vi "GrabCallBackThread_FullFeatures.vi"(11 "Error IN":errorcluster) -> (15 "Error OUT":errorcluster)   [LabVIEW 2014]
uses:
  <vilib>/addons/PixeLINK/Low Level Functions/TRANSLATION.llb/TDPU-Translation-CallBackFlags.ctl
  <vilib>/addons/PixeLINK/Low Level Functions/TRANSLATION.llb/TDPU-Translation-CallbacksInfo.ctl
  <vilib>/addons/PixeLINK/Low Level Functions/ACQUISITION.llb/TDPU-Acquisition-Frame_Desc.ctl
  <vilib>/addons/PixeLINK/Low Level Functions/TRANSLATION.llb/TDPU-Translation-PixelFormat.ctl
  <vilib>/addons/PixeLINK/Low Level Functions/ACQUISITION.llb/TDPU-Acquisition-StreamState.ctl
  <vilib>/addons/PixeLINK/Low Level Functions/CAMERA_FEATURES.llb/TDPU-CameraFeatures-FeatureIds.ctl
  <vilib>/addons/PixeLINK/Low Level Functions/CAMERA_FEATURES.llb/TDPU-CameraFeatures-FeatureFlags.ctl
  PxLLabVIEW.dll
panel:
  in  "Trig":u16(ring) items=["Freerun", "Software", "Hardware"]
  in  "Stop Processing Events":bool
  out "Loop info":string
  in  "Exposure time":dbl=7e-05 min=7e-05 max=5.0
  out "Intensity Graph":u16[][](graph)
  out "Frame Number":u32
  out "Missed Frames":u32
  out "FrameData_FORMAT":T1 items=["PIXEL_FORMAT_MONO8", "PIXEL_FORMAT_MONO16", "PIXEL_FORMAT_YUV422", "PIXEL_FORMAT_BAYER8", "PIXEL_FORMAT_BAYER16", "PIXEL_FORMAT_RGB24", "PIXEL_FORMAT_RGB48"]
  out "FRAME_DESC":T2 {"PixelAddressingMode"."fValue" format="%.2f"; "Rotate"."fValue" format="%.2f"; "WhiteShading"."fBlueGain" format="%.2f"; "WhiteShading"."fGreenGain" format="%.2f"; "WhiteShading"."fRedGain" format="%.2f"; "AutoROI"."fHeight" format="%.2f"; "AutoROI"."fWidth" format="%.2f"; "AutoROI"."fTop" format="%.2f"; "AutoROI"."fLeft" format="%.2f"; "ExtendedShutter"."fKneePoint" format="%.2f"; "PixelFormat"."fValue" format="%.2f"; "PixelAddressingValue"."fValue" format="%.2f"; "Flip"."fVertical" format="%.2f"; "Flip"."fHorizontal" format="%.2f"; "ROI"."fHeight" format="%.2f"; "ROI"."fWidth" format="%.2f"; "ROI"."fTop" format="%.2f"; "ROI"."fLeft" format="%.2f"; "FrameRate"."fValue" format="%.2f"; "GPIO"."fParameter3" format="%.2f"; "GPIO"."fParameter2" format="%.2f"; "GPIO"."fParameter1" format="%.2f"; "GPIO"."fPolarity" format="%.2f"; "GPIO"."fMode" format="%.2f"; "OpticalFilter"."fValue" format="%.2f"; "Tilt"."fValue" format="%.2f"; "Pan"."fValue" format="%.2f"; "Zoom"."fValue" format="%.2f"; "Trigger"."fParameter" format="%.2f"; "Trigger"."fDelay" format="%.2f"; "Trigger"."fPolarity" format="%.2f"; "Trigger"."fType" format="%.2f"; "Trigger"."fMode" format="%.2f"; "Temperature"."fValue" format="%.2f"; "Focus"."fValue" format="%.2f"; "Iris"."fValue" format="%.2f"; "Gain"."fValue" format="%.2f"; "Shutter"."fValue" format="%.2f"; "Gamma"."fValue" format="%.2f"; "Saturation"."fValue" format="%.2f"; "Hue"."fValue" format="%.2f"; "WhiteBalance"."fValue" format="%.2f"; "Sharpness"."fValue" format="%.2f"; "AutoExposure"."fValue" format="%.2f"; "Brightness"."fValue" format="%.2f"; "fFrameTime" format="%.2f"}
  in  "CallbacksInfo IN":T3 {"uOverlayUse" items=["OVERLAY_PREVIEW             0x01", "OVERLAY_FORMAT_IMAGE  0x02", "OVERLAY_FORMAT_CLIP     0x04", "OVERLAY_FRAME                 0x08"]}
  out "FrameData":u8[](array[numeric]) format="%.0x"
  in  "Path IN":path
  in  "hCamera IN":u32
  in  "uOverlayUse IN":T4 items=["OVERLAY_PREVIEW             0x01", "OVERLAY_FORMAT_IMAGE  0x02", "OVERLAY_FORMAT_CLIP     0x04", "OVERLAY_FRAME                 0x08"]
  in  "Occurrence IN":refnum<k4>
  in  "Stop":bool
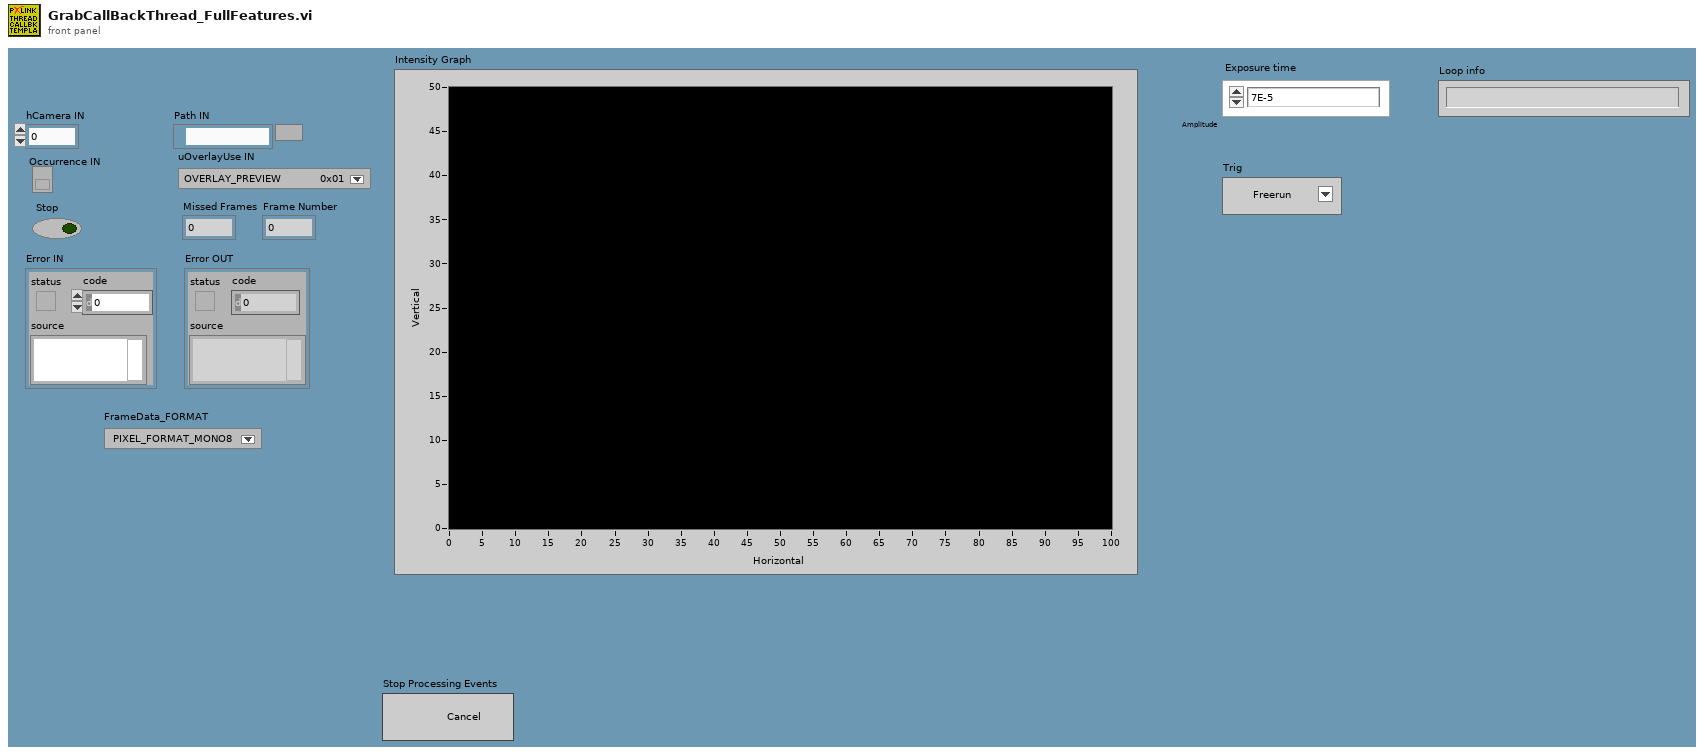
[diagram p1: front panel]
types:
  T1 = typedef "TDPU-Translation-PixelFormat.ctl" = u32
  T2 = typedef "TDPU-Acquisition-Frame_Desc.ctl" = cluster{"uSize":u32, "fFrameTime":dbl, "uFrameNumber":u32, "Brightness":cluster{"fValue":dbl}, "AutoExposure":cluster{"fValue":dbl}, "Sharpness":cluster{"fValue":dbl}, "WhiteBalance":cluster{"fValue":dbl}, "Hue":cluster{"fValue":dbl}, "Saturation":cluster{"fValue":dbl}, "Gamma":cluster{"fValue":dbl}, "Shutter":cluster{"fValue":dbl}, "Gain":cluster{"fValue":dbl}, "Iris":cluster{"fValue":dbl}, "Focus":cluster{"fValue":dbl}, "Temperature":cluster{"fValue":dbl}, "Trigger":cluster{"fMode":dbl, "fType":dbl, "fPolarity":dbl, "fDelay":dbl, "fParameter":dbl}, "Zoom":cluster{"fValue":dbl}, "Pan":cluster{"fValue":dbl}, "Tilt":cluster{"fValue":dbl}, "OpticalFilter":cluster{"fValue":dbl}, "GPIO":cluster{"fMode":dbl[], "fPolarity":dbl[], "fParameter1":dbl[], "fParameter2":dbl[], "fParameter3":dbl[]}, "FrameRate":cluster{"fValue":dbl}, "ROI":cluster{"fLeft":dbl, "fTop":dbl, "fWidth":dbl, "fHeight":dbl}, "Flip":cluster{"fHorizontal":dbl, "fVertical":dbl}, "PixelAddressingValue":cluster{"fValue":dbl}, "PixelFormat":cluster{"fValue":dbl}, "ExtendedShutter":cluster{"fKneePoint":dbl[]}, "AutoROI":cluster{"fLeft":dbl, "fTop":dbl, "fWidth":dbl, "fHeight":dbl}, "WhiteShading":cluster{"fRedGain":dbl, "fGreenGain":dbl, "fBlueGain":dbl}, "Rotate":cluster{"fValue":dbl}, "PixelAddressingMode":cluster{"fValue":dbl}}
  T3 = typedef "TDPU-Translation-CallbacksInfo.ctl" = cluster{"Occurrence":refnum<k4>, "hCamera":u32, "uOverlayUse":T4, "Path":path, "bGetClip":bool, "uNumberofFrameCaptured":u32, "error (Get Clip) ":errorcluster, "TerminationOccurence":refnum<k4>, "PDS Clip Path":path, "AVI Clip Path":path}
  T4 = typedef "TDPU-Translation-CallBackFlags.ctl" = u32
  T5 = typedef "TDPU-Acquisition-StreamState.ctl" = u32
  T6 = typedef "TDPU-CameraFeatures-FeatureFlags.ctl" = u32
  T7 = typedef "TDPU-CameraFeatures-FeatureIds.ctl" = u32
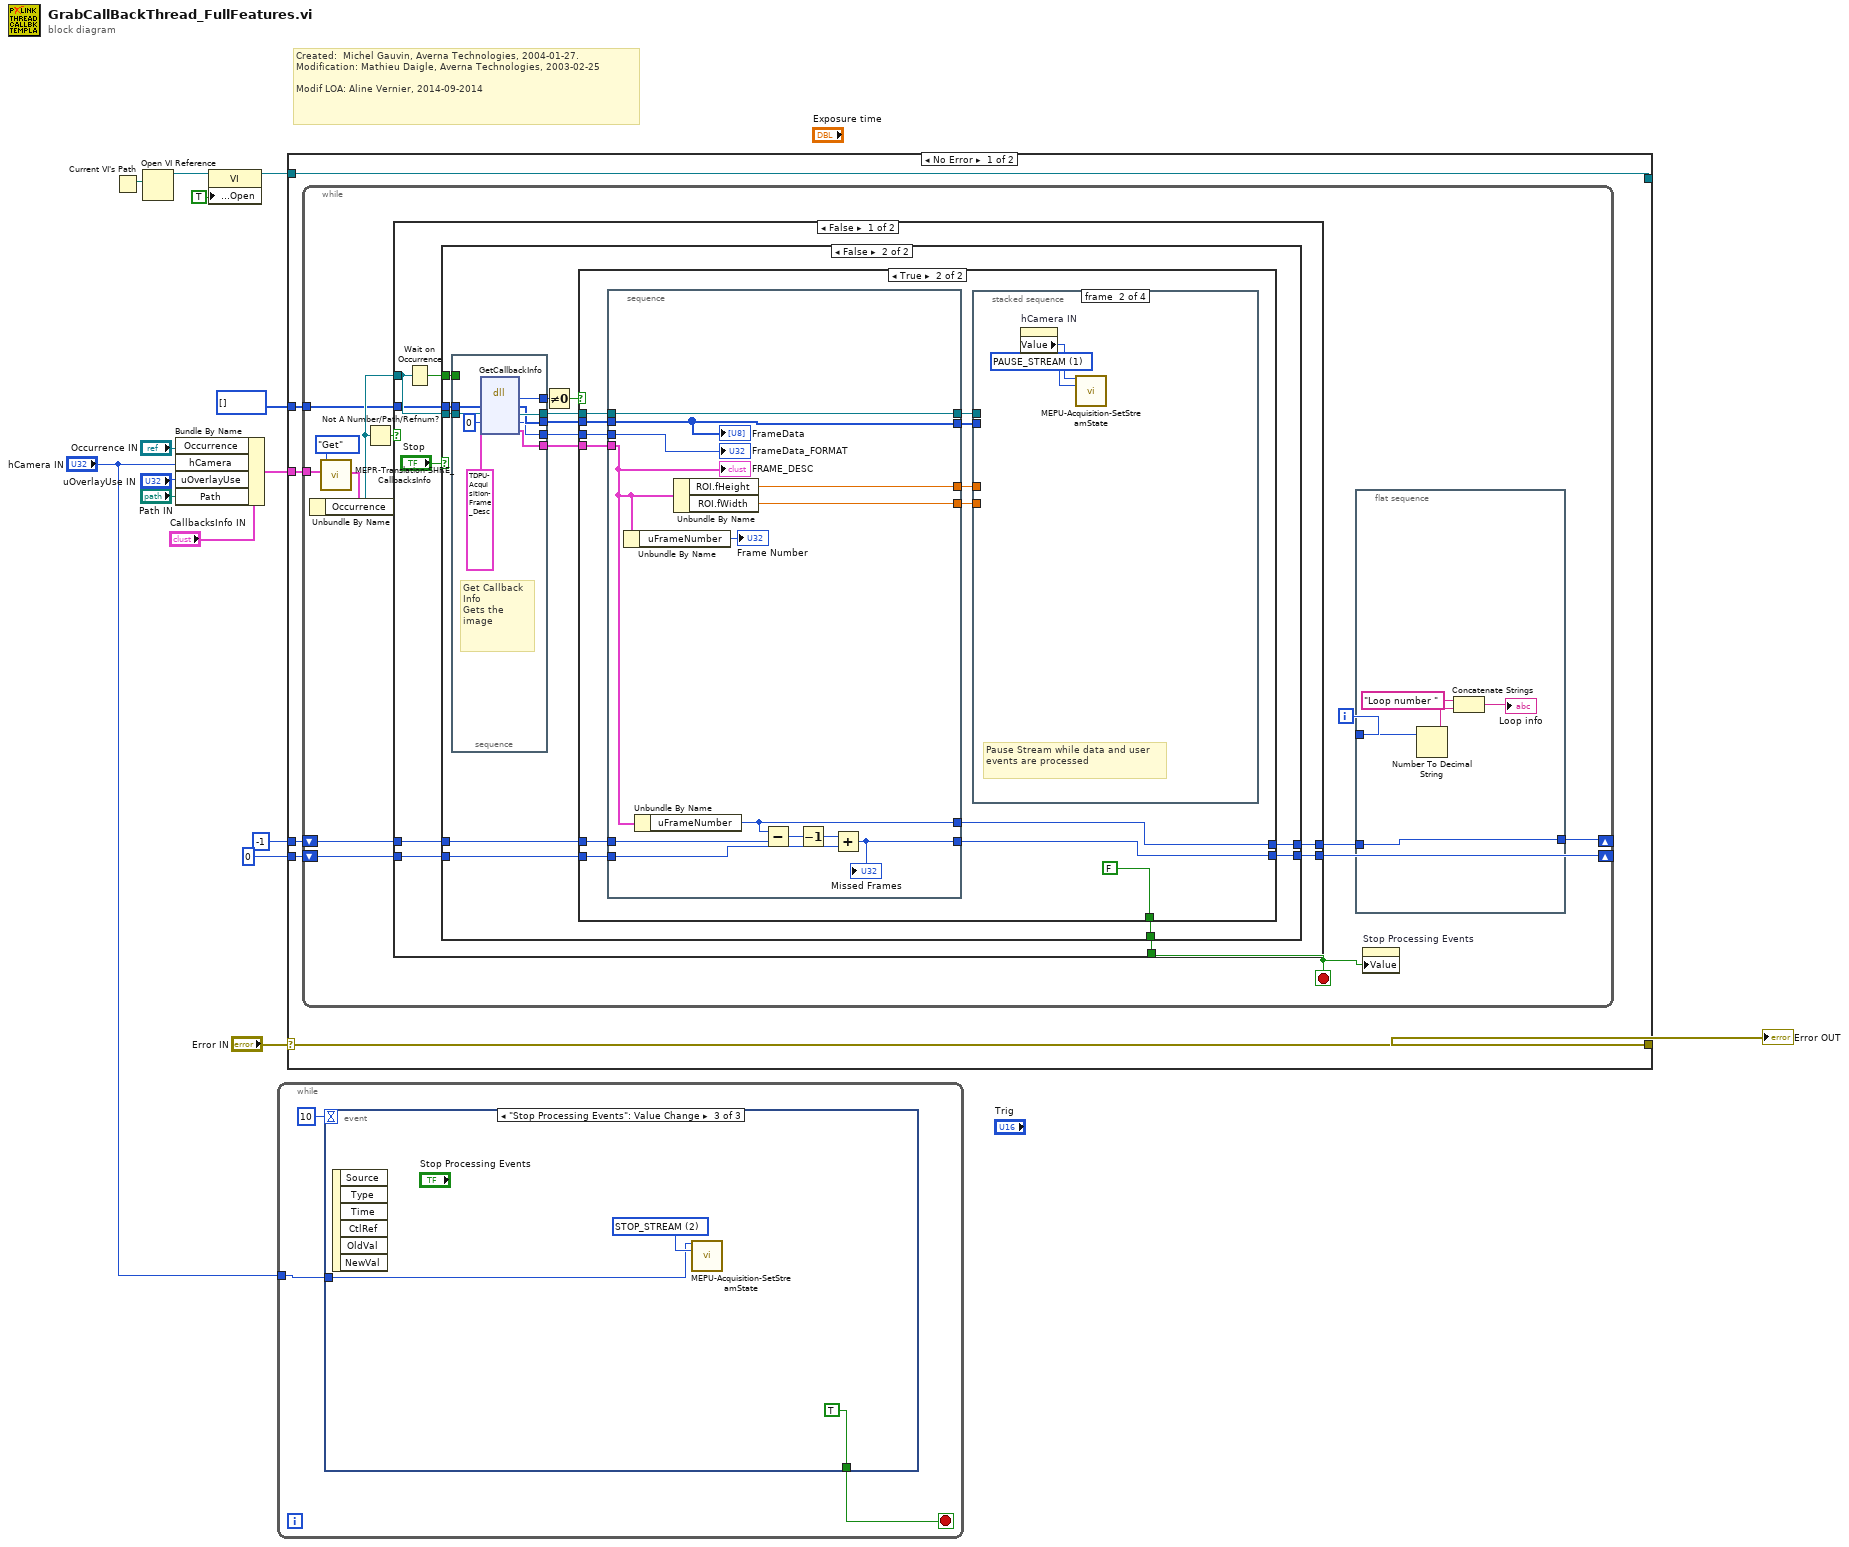
[diagram p0: block diagram]
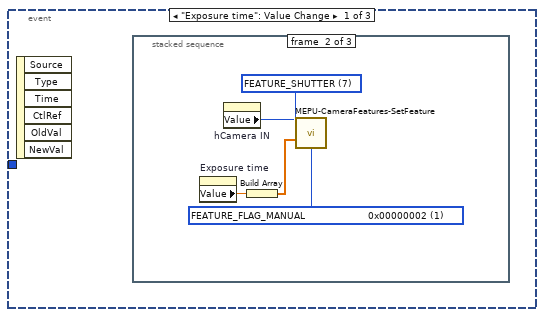
[diagram p2: hidden frame]
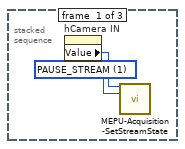
[diagram p3: hidden frame]
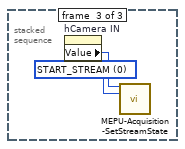
[diagram p4: hidden frame]
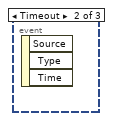
[diagram p5: hidden frame]
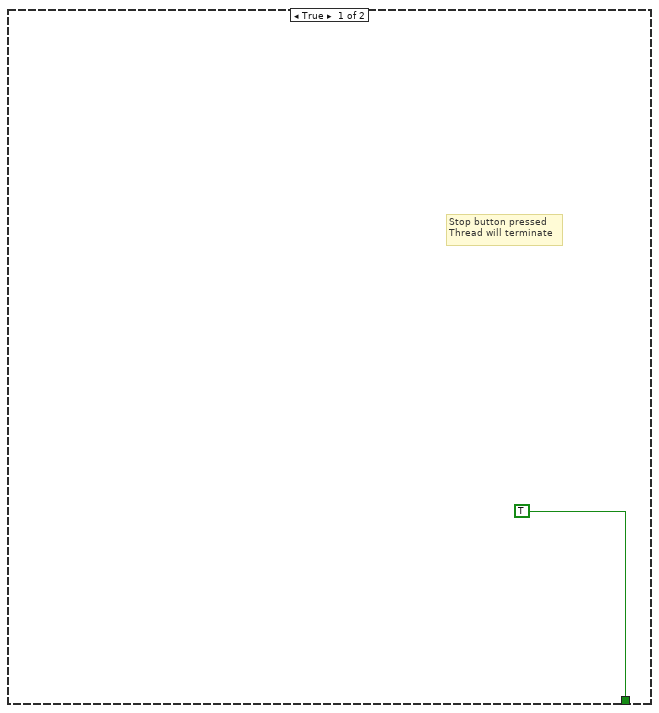
[diagram p6: hidden frame]
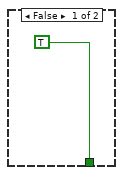
[diagram p7: hidden frame]
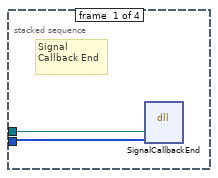
[diagram p8: hidden frame]
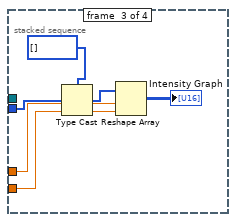
[diagram p9: hidden frame]
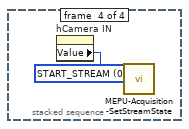
[diagram p10: hidden frame]
diagram:
  # "Created:  Michel Gauvin, Averna Technologies, 2004-01-27.\nModification: Mathieu Daigle, Averna Technologies, 2003-02-25\n\nModif LOA: Aline Vernier, 2014-09-2014"
  n1 = Current VI's Path() -> (path=w14:path)
  n2 = Open VI Reference(vi path=w14) -> (vi reference=w13:refnum<vi>)  [unwired: 5 in, 1 out]
  n3 = Bundle By Name(cluster="CallbacksInfo IN", "Occurrence"="Occurrence IN", "hCamera"="hCamera IN", "uOverlayUse"="uOverlayUse IN", "Path"="Path IN") -> (w9:T3)
  n4 = property class="VI"(reference=w13, "Front Panel Window:Open"=TRUE) -> (reference out=w11:refnum<vi>)  [unwired: 1 in, 1 out]
  n5 = while {
    tunnel: "hCamera IN" -> [w17]
    stop <- w18 stop-if-true
    n6 = event shown="[2] \"Stop Processing Events\": Value Change" {
      selector: _ -> [_ _ _]
      dyn-events: _ -> [_ _ _]
      timeout: 10 -> [_ _ _]
      tunnel: [_ _ TRUE] -> w18
      tunnel: w17 -> [_ _ w28]
      event "Exposure time": Value Change {
        n7 = event-data() -> ()  [unwired: 1 in, 6 out]
        n8 = stacked-sequence {
          frame #0 {
            w20 = T5 1 items=["START_STREAM", "PAUSE_STREAM", "STOP_STREAM"] ("uStreamState IN")
            n9 = property on="hCamera IN" class="DigNum (strict)"() -> ("Value"=w19:u32)  [unwired: 2 in, 2 out]
            n10 = call <vilib>:"MEPU-Acquisition-SetStreamState.vi"("hCamera IN"=w19, "uStreamState IN"=w20) -> ()  [unwired: 12 in, 2 out]
          }
          frame #1 {
            w25 = T6 1 items=["FEATURE_FLAG_PRESENCE                 0x00000001", "FEATURE_FLAG_MANUAL                     0x00000002", "FEATURE_FLAG_AUTO                         0x00000004", "FEATURE_FLAG_ONEPUSH                   0x00000008", "FEATURE_FLAG_OFF                            0x00000010", "FEATURE_FLAG_DESC_SUPPORTED    0x00000020", "FEATURE_FLAG_READ_ONLY               0x00000040"] ("uFlags IN")
            w22 = T7 7 items=["FEATURE_BRIGHTNESS", "FEATURE_EXPOSURE", "FEATURE_SHARPNESS", "FEATURE_WHITE_BAL", "FEATURE_HUE", "FEATURE_SATURATION", "FEATURE_GAMMA", "FEATURE_SHUTTER", "FEATURE_GAIN", "FEATURE_IRIS", "FEATURE_FOCUS", "FEATURE_TEMPERATURE", "FEATURE_TRIGGER", "FEATURE_ZOOM", "FEATURE_PAN", "FEATURE_TILT", "FEATURE_OPT_FILTER", "FEATURE_GPIO", "FEATURE_FRAME_RATE", "FEATURE_ROI", "FEATURE_FLIP", "FEATURE_PIXEL_ADDRESSING", "FEATURE_PIXEL_FORMAT", "FEATURE_EXTENDED_SHUTTER", "FEATURE_AUTO_ROI", "FEATURE_LOOKUP_TABLE", "FEATURE_MEMORY_CHANNEL", "FEATURE_WHITE_SHADING", "FEATURE_ROTATE", "FEATURE_IMAGER_CLK_DIVISOR", "FEATURE_TRIG_WITH_CNTRLD_LIGHT", "FEATURE_MAX_PIXEL_SIZE"] ("uFeatureId IN")
            n11 = property on="Exposure time" class="DigNum (strict)"() -> ("Value"=w23:dbl)  [unwired: 2 in, 2 out]
            n12 = property on="hCamera IN" class="DigNum (strict)"() -> ("Value"=w21:u32)  [unwired: 2 in, 2 out]
            n13 = Build Array(w23) -> (w24:dbl[])
            n14 = call <vilib>:"MEPU-CameraFeatures-SetFeature.vi"("hCamera IN"=w21, "uFeatureId IN"=w22, "uFlags IN"=w25, "pParms IN"=w24) -> ()  [unwired: 9 in, 3 out]
          }
          frame #2 {
            w27 = T5 0 items=["START_STREAM", "PAUSE_STREAM", "STOP_STREAM"] ("uStreamState IN")
            n15 = property on="hCamera IN" class="DigNum (strict)"() -> ("Value"=w26:u32)  [unwired: 2 in, 2 out]
            n16 = call <vilib>:"MEPU-Acquisition-SetStreamState.vi"("hCamera IN"=w26, "uStreamState IN"=w27) -> ()  [unwired: 12 in, 2 out]
          }
        }
      }
      event Timeout {
        n17 = event-data() -> ()  [unwired: 1 in, 3 out]
      }
      event "Stop Processing Events": Value Change {
        w29 = T5 2 items=["START_STREAM", "PAUSE_STREAM", "STOP_STREAM"] ("uStreamState IN")
        n18 = event-data() -> ()  [unwired: 1 in, 6 out]
        n19 = call <vilib>:"MEPU-Acquisition-SetStreamState.vi"("hCamera IN"=w28, "uStreamState IN"=w29) -> ()  [unwired: 12 in, 2 out]
      }
    }
  }
  n20 = case shown="No Error" "Error IN" {
    selector: "Error IN" -> [w36 w129]
    tunnel: [w36 w129] -> w15
    tunnel: w11 -> [w35 w128]
    tunnel: [w35 w128] -> _
    tunnel: w9 -> [w34 _]
    tunnel: u8[] [] -> [w33 _]
    tunnel: u32 0 -> [w32 _]
    tunnel: -1 -> [w31 _]
    frame No Error {
      n21 = while {
        tunnel: w34 -> [w48]
        tunnel: w33 -> [w44]
        shift-right: [w39] -> _
        shift-left: w31 -> [w43]
        shift-right: [w41] -> _
        shift-left: w32 -> [w42]
        i -> [w38]
        stop <- w37 stop-if-true
        n22 = call <vilib>:"MEPR-Translation-SHRE_CallbacksInfo.vi"("Action"=enum16{"Get", "Clear", "Init", "Set"}."Get", "CallbackInfo IN"=w48) -> ("CallbackInfo OUT"=w47:T3)  [unwired: 15 in, 2 out]
        n23 = Unbundle By Name(w47) -> ("Occurrence"=w46:refnum<k4>)
        n24 = Not A Number/Path/Refnum?(number/path/refnum=w46) -> (NaN/Path/Refnum?=w49:bool)
        n25 = case shown="False" w49 {
          selector: w49 -> [_ w127]
          tunnel: w46 -> [w63 _]
          tunnel: [w55 w127] -> w37
          tunnel: w44 -> [w60 _]
          tunnel: [w59 _] -> w40
          tunnel: w43 -> [w58 _]
          tunnel: w42 -> [w57 _]
          tunnel: [w56 _] -> w41
          frame False {
            n26 = Wait on Occurrence(2:w63) -> (0:w62:bool)  [unwired: 2 in]
            n27 = case shown="False" "Stop" {
              tunnel: w63 -> [_ w78]
              tunnel: w62 -> [_ w77]
              tunnel: w60 -> [_ w74]
              tunnel: [_ w71] -> w59
              tunnel: w58 -> [_ w70]
              tunnel: w57 -> [_ w69]
              tunnel: [_ w68] -> w56
              tunnel: [TRUE w65] -> w55
              frame True {
                # "Stop button pressed\nThread will terminate"
              }
              frame False {
                n28 = stacked-sequence {
                  tunnel: w78 -> [w125]
                  tunnel: [w126] -> w66
                  tunnel: w77 -> [_]
                  tunnel: [w123] -> w76
                  tunnel: [w124] -> w75
                  tunnel: w74 -> [w122]
                  tunnel: [w119] -> w73
                  tunnel: [w118] -> w72
                  frame #0 {
                    # "Get Callback Info\nGets the image"
                    n29 = dll-call lib="PxLLabVIEW.dll" fn="GetCallbackInfo"("output param"=w122, "Occurrence"=w125, "pDataFormat"=u32 0, "FRAME_DESC"=T2 {"uSize"=0, "fFrameTime"=0.0, "uFrameNumber"=0, "Brightness"={"fValue"=0.0}, "AutoExposure"={"fValue"=0.0}, "Sharpness"={"fValue"=0.0}, "WhiteBalance"={"fValue"=0.0}, "Hue"={"fValue"=0.0}, "Saturation"={"fValue"=0.0}, "Gamma"={"fValue"=0.0}, "Shutter"={"fValue"=0.0}, "Gain"={"fValue"=0.0}, "Iris"={"fValue"=0.0}, "Focus"={"fValue"=0.0}, "Temperature"={"fValue"=0.0}, "Trigger"={"fMode"=0.0, "fType"=0.0, "fPolarity"=0.0, "fDelay"=0.0, "fParameter"=0.0}, "Zoom"={"fValue"=0.0}, "Pan"={"fValue"=0.0}, "Tilt"={"fValue"=0.0}, "OpticalFilter"={"fValue"=0.0}, "GPIO"={"fMode"=[], "fPolarity"=[], "fParameter1"=[], "fParameter2"=[], "fParameter3"=[]}, "FrameRate"={"fValue"=0.0}, "ROI"={"fLeft"=0.0, "fTop"=0.0, "fWidth"=0.0, "fHeight"=0.0}, "Flip"={"fHorizontal"=0.0, "fVertical"=0.0}, "PixelAddressingValue"={"fValue"=0.0}, "PixelFormat"={"fValue"=0.0}, "ExtendedShutter"={"fKneePoint"=[]}, "AutoROI"={"fLeft"=0.0, "fTop"=0.0, "fWidth"=0.0, "fHeight"=0.0}, "WhiteShading"={"fRedGain"=0.0, "fGreenGain"=0.0, "fBlueGain"=0.0}, "Rotate"={"fValue"=0.0}, "PixelAddressingMode"={"fValue"=0.0}}) -> (w126:i32, "output param"=w123:u8[], "Occurrence"=w124:refnum<k4>, "pDataFormat"=w118:u32, "FRAME_DESC"=w119:T2)  [unwired: 3 in, 2 out]
                  }
                }
                n30 = Not Equal To 0?(x=w66) -> (x != 0?=w67:bool)
                n31 = case shown="True" w67 {
                  tunnel: w76 -> [_ w91]
                  tunnel: w75 -> [_ w90]
                  tunnel: w73 -> [_ w89]
                  tunnel: w72 -> [_ w88]
                  tunnel: [_ w83] -> w71
                  tunnel: w70 -> [_ w87]
                  tunnel: w69 -> [_ w86]
                  tunnel: [_ w85] -> w68
                  tunnel: [TRUE FALSE] -> w65
                  frame False {
                  }
                  frame True {
                    n32 = stacked-sequence {
                      tunnel: w90 -> [w117]
                      tunnel: [w117] -> w92
                      tunnel: w91 -> [w107]
                      tunnel: w89 -> [w109]
                      tunnel: w88 -> [w110]
                      tunnel: [w116] -> w83
                      tunnel: w87 -> [w115]
                      tunnel: w86 -> [w112]
                      tunnel: [w111] -> w85
                      tunnel: [w107] -> w82
                      tunnel: [w106] -> w81
                      tunnel: [w105] -> w80
                      frame #0 {
                        n33 = Unbundle By Name(w109) -> ("uFrameNumber"=→"Frame Number":u32)
                        n34 = Unbundle By Name(w109) -> ("uFrameNumber"=w116:u32)
                        n35 = Unbundle By Name(w109) -> ("ROI.fHeight"=w106:dbl, "ROI.fWidth"=w105:dbl)
                        n36 = Subtract(x=w116, y=w115) -> (x-y=w114:u32)
                        n37 = Decrement(x=w114) -> (x-1=w113:u32)
                        n38 = Add(x=w113, y=w112) -> (x+y=w111:u32)
                        "Missed Frames" <- w111
                        "FrameData" <- w107
                        "FRAME_DESC" <- w109
                        "FrameData_FORMAT" <- w110
                      }
                    }
                    n39 = stacked-sequence {
                      tunnel: w92 -> [w94 _ _ _]
                      tunnel: w82 -> [w93 _ w101 _]
                      tunnel: w81 -> [_ _ w97 _]
                      tunnel: w80 -> [_ _ w99 _]
                      frame #0 {
                        # "Signal Callback End"
                        n40 = dll-call lib="PxLLabVIEW.dll" fn="SignalCallbackEnd"("Occurrence"=w94, "Data"=w93) -> ()  [unwired: 6 in, 2 out]
                      }
                      frame #1 {
                        w95 = T5 1 items=["START_STREAM", "PAUSE_STREAM", "STOP_STREAM"] ("uStreamState IN")
                        # "Pause Stream while data and user events are processed"
                        n41 = property on="hCamera IN" class="DigNum (strict)"() -> ("Value"=w96:u32)  [unwired: 2 in, 2 out]
                        n42 = call <vilib>:"MEPU-Acquisition-SetStreamState.vi"("hCamera IN"=w96, "uStreamState IN"=w95) -> ()  [unwired: 12 in, 2 out]
                      }
                      frame #2 {
                        n43 = Type Cast(type=u16[] [] ("output param"), x=w101) -> (*(type *) &x=w100:u16[])
                        n44 = Reshape Array(w100, w97, w99) -> (→"Intensity Graph":u16[][])
                      }
                      frame #3 {
                        w103 = T5 0 items=["START_STREAM", "PAUSE_STREAM", "STOP_STREAM"] ("uStreamState IN")
                        n45 = property on="hCamera IN" class="DigNum (strict)"() -> ("Value"=w104:u32)  [unwired: 2 in, 2 out]
                        n46 = call <vilib>:"MEPU-Acquisition-SetStreamState.vi"("hCamera IN"=w104, "uStreamState IN"=w103) -> ()  [unwired: 12 in, 2 out]
                      }
                    }
                  }
                }
              }
            }
          }
          frame True {
          }
        }
        n47 = flat-sequence {
          tunnel: w40 -> [w54]
          tunnel: [w54] -> w39
          tunnel: w38 -> [w53]
          frame #0 {
            n48 = Number To Decimal String(number=w53) -> (decimal integer string=w51:string)  [unwired: 1 in]
            n49 = Concatenate Strings("Loop number " ("string"), w51) -> (→"Loop info":string)
          }
        }
        n50 = property on="Stop Processing Events" class="Bool (strict)"("Value"=w37) -> ()  [unwired: 2 in, 2 out]
      }
    }
    frame Error {
    }
  }
  "Error OUT" <- w15
